vi "CloseQueue.vi"(8 "error in (no error)":errorcluster, 11 "ModuleAdmin In":refnum<class "ModuleAdmin.lvclass">) -> (0 "error out":errorcluster, 3 "ModuleAdminOut":refnum<class "ModuleAdmin.lvclass">)   [LabVIEW 2018, in "ModuleAdmin.lvlib" / "ModuleAdmin.lvclass"]
uses:
  ModuleAdmin.lvclass
  ModuleAdmin.lvclass/ModuleAdmin.ctl
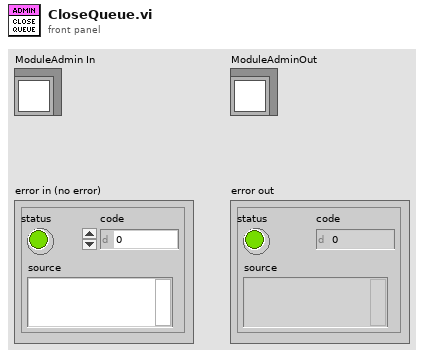
[diagram p1: front panel]
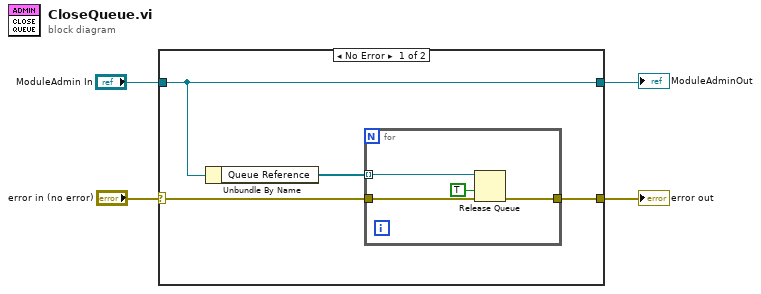
[diagram p0: block diagram]
diagram:
  n1 = case shown="No Error" "error in (no error)" {
    selector: "error in (no error)" -> [w8 w13]
    tunnel: "ModuleAdmin In" -> [w5 w14]
    tunnel: [w5 w14] -> w2
    tunnel: [w7 w13] -> w1
    frame No Error {
      n2 = Unbundle By Name(w5) -> ("Queue Reference"=w6:refnum<queue>[])
      n3 = for {
        tunnel: w8 -> [w12]
        tunnel: [w11] -> w7
        tunnel: w6 -> [w10] mode=indexing
        n4 = Release Queue(queue=w10, force destroy? (F)=TRUE, error in (no error)=w12) -> (error out=w11:errorcluster)  [unwired: 2 out]
      }
    }
    frame Error {
    }
  }
  "error out" <- w1
  "ModuleAdminOut" <- w2
